vi "example.vi"() -> ()   [LabVIEW 2013]
panel:
  out "qual error %":dbl format="%_3g"
  out "flow error %":dbl format="%#_2g"
  out "runoff error %":dbl format="%#_1g"
  out "Waveform Chart":dbl[](graph)
  in  "SWMM Input File (.inp)":path
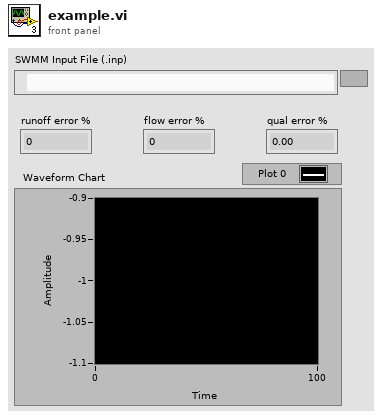
[diagram p1: front panel]
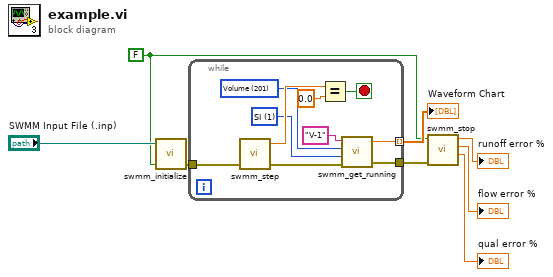
[diagram p0: block diagram]
diagram:
  w4 = FALSE ("Success msg?")
  n1 = call "swmm_initialize.vi"("Success msg?"=w4, "SWMM Input File (.inp)"="SWMM Input File (.inp)") -> ("error out"=w7:errorcluster)  [unwired: 3 in]
  n2 = while {
    tunnel: w7 -> [w15]
    tunnel: [w14] -> w6 mode=indexing
    tunnel: [w12] -> w5
    stop <- w17 stop-if-true
    w9 = 1 items=["US", "SI"] ("Unit system")
    w10 = 201 items=["Depth"=200, "Volume"=201, "Flow"=202, "Setting"=203, "Froude"=204, "Inflow"=205, "Flooding"=206, "Precipitation"=207, "Runoff"=208] ("Attribute")
    n3 = call "swmm_step.vi"("error in (no error)"=w15) -> ("error out"=w13:errorcluster, "new_elapsed_time"=w16:dbl)  [unwired: 3 in]
    n4 = Equal?(x=w16, y=0.0) -> (x = y?=w17:bool)
    n5 = call "swmm_get_running.vi"("error in"=w13, "Unit system"=w9, "Attribute"=w10, "object_id"="V-1") -> ("error out"=w12:errorcluster, "value"=w14:dbl)  [unwired: 1 in]
  }
  "Waveform Chart" <- w6
  n6 = call "swmm_stop.vi"("error in"=w5, "Success msg?"=w4) -> ("qual error"=→"qual error %":dbl, "flow error"=→"flow error %":dbl, "runoff error"=→"runoff error %":dbl)  [unwired: 2 in, 1 out]
